vi "Colorbar2001.vi"   [LabVIEW 2013]
uses:
  <vilib>/Heliosphere Research LLC/Advanced Plotting Toolkit/Advanced Plotting Toolkit.lvlib
types:
  T1 = typedef "Advanced Plotting Toolkit.lvlib/PlotID.ctl" = i32
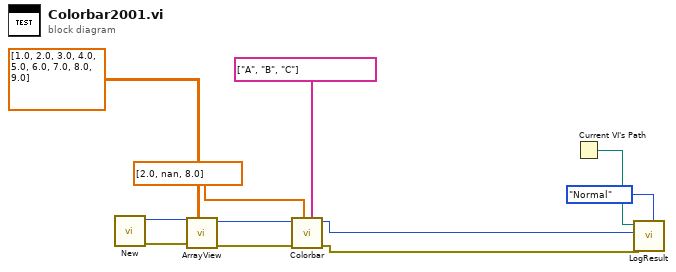
[diagram p0: block diagram]
diagram:
  n1 = call <vilib>:"New.vi"() -> ("error out"=w10:errorcluster, "Plot ID"=w9:T1)  [unwired: 10 in]
  n2 = call <vilib>:"ArrayView.vi"("Data"=dbl[][] [[1.0, 2.0, 3.0], [4.0, 5.0, 6.0], [7.0, 8.0, 9.0]], "error in (no error)"=w10, "Plot ID"=w9) -> ("error out"=w6:errorcluster, "Plot ID Out"=w7:T1)  [unwired: 7 in]
  n3 = call <vilib>:"Colorbar.vi"("Tick Labels"=string[] ["A", "B", "C"], "Ticks"=dbl[] [2.0, nan, 8.0], "error in (no error)"=w6, "Plot ID"=w7) -> ("error out"=w5:errorcluster, "Plot ID Out"=w4:T1)  [unwired: 6 in]
  n4 = Current VI's Path() -> (path=w11:path)
  n5 = call "LogResult.vi"("Mode"=enum16{"Normal", "Expected Failure"}."Normal", "Test Result"=w5, "Test Artifact"=w4, "VI Path"=w11) -> ()  [unwired: 8 in]
